vi "Comma Separated Strings to String Array.vi"(1 "Comma Separated Strings":string) -> (15 "String Array":string[](array[string]))   [LabVIEW 2015, in "RT Management.lvlib" / "Module Detection.lvclass"]
uses:
  Module Detection.lvclass
  <vilib>/regexp/Match Regular Expression.xnode
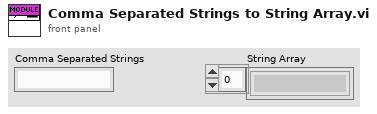
[diagram p1: front panel]
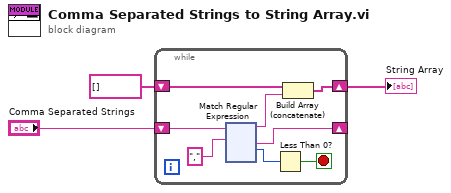
[diagram p0: block diagram]
diagram:
  n1 = while {
    shift-right: [w7] -> w3
    shift-left: string[] [] -> [w8]
    shift-right: [w5] -> _
    shift-left: "Comma Separated Strings" -> [w11]
    stop <- w6 stop-if-true
    n2 = xnode "Match Regular Expression"("input string"=w11, "regular expression"=",") -> ("before match"=w4:string, "after match"=w5:string, "offset past match"=w9:i32)  [unwired: 4 in, 2 out]
    n3 = Less Than 0?(x=w9) -> (x < 0?=w6:bool)
    n4 = Build Array (concatenate)(w8, w4) -> (w7:string[])
  }
  "String Array" <- w3
